vi "pointer.permute.advanced copy.vi"(8 "error in (no error)":errorcluster, 11 "TestCase in":refnum<class "TestCase.Pointer.lvclass">) -> (0 "error out":errorcluster, 2 "pass?":bool, 3 "TestCase out":refnum<class "TestCase.Pointer.lvclass">)   [LabVIEW 2016, in "TestCase.Pointer.lvclass"]
uses:
  TestCase.Pointer.lvclass
  TestCase.Pointer.lvclass/TestCase.Pointer.ctl
  Source/Classes/Pointer/Memory.Pointer.Write.0D.DBL.vi
  Source/Classes/Pointer/Memory.Pointer.Read.0D.U8.vi
  Source/Classes/Pointer/Memory.Pointer.Read.0D.U16.vi
  Source/Classes/Pointer/Memory.Pointer.Read.0D.U32.vi
  Source/Classes/Pointer/Memory.Pointer.Read.0D.U64.vi
  Source/Classes/Pointer/Memory.Pointer.lvclass
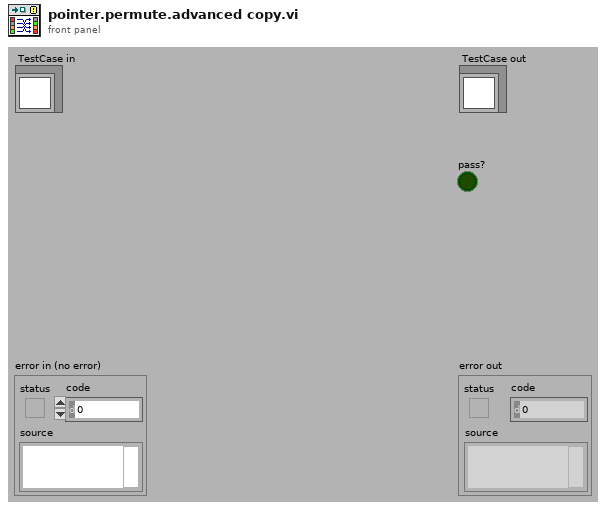
[diagram p1: front panel]
types:
  T1 = enum16{"big-endian, network order", "native, host order", "little-endian"}
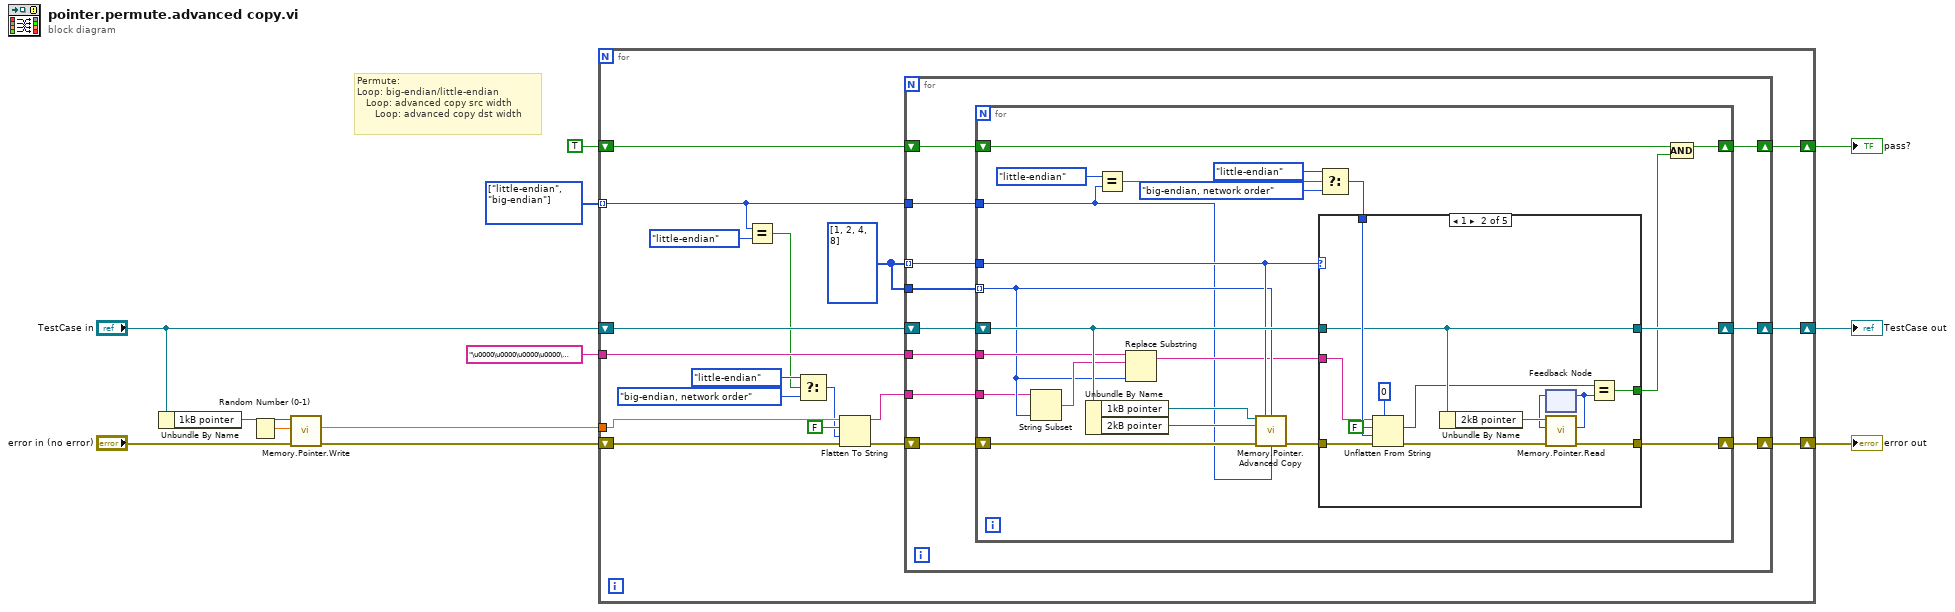
[diagram p0: block diagram]
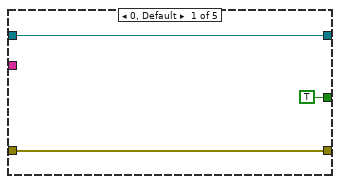
[diagram p2: hidden frame]
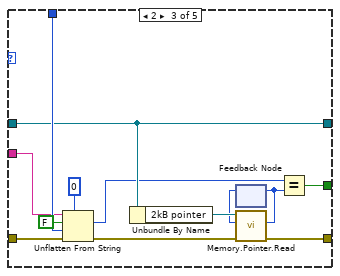
[diagram p3: hidden frame]
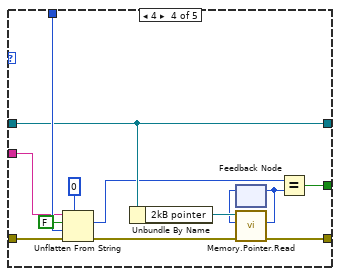
[diagram p4: hidden frame]
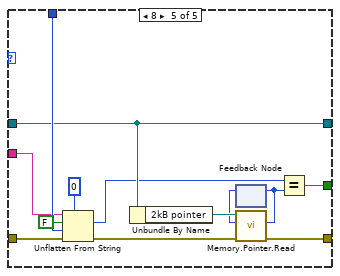
[diagram p5: hidden frame]
diagram:
  w10 = enum16{"big-endian", "little-endian"}[] [enum."little-endian", enum."big-endian"] items=["big-endian", "little-endian"] ("byte order (big-endian)")
  # "Permute:\nLoop: big-endian/little-endian\n   Loop: advanced copy src width\n      Loop: advanced copy dst width"
  n1 = Unbundle By Name("TestCase in") -> ("1kB pointer"=w9:refnum<class "Memory.Pointer.lvclass">)
  n2 = Random Number (0-1)() -> (number: 0 to 1=w8:dbl)
  n3 = call-poly "Memory.Pointer.Write.vi"("error in (no error)"="error in (no error)", "value"=w8, "Pointer in"=w9) -> ("error out"=w1:errorcluster, "value"=w2:dbl)  [unwired: 5 in, 2 out]
  n4 = for {
    shift-right: [w29] -> w12
    shift-left: w1 -> [w22]
    shift-right: [w28] -> w11
    shift-left: "TestCase in" -> [w30]
    tunnel: w10 -> [w13] mode=indexing
    shift-right: [w25] -> w4
    shift-left: TRUE -> [w26]
    tunnel: "\u0000\u0000\u0000\u0000\u0000\u0000\u0000\u0000" -> [w24]
    tunnel: w2 -> [w19]
    w27 = u64[] [1, 2, 4, 8] ("dst width")
    n5 = Equal?(x=w13, y=enum16{"big-endian", "little-endian"}."little-endian" ("byte order (big-endian)")) -> (x = y?=w15:bool)
    n6 = Select(t=T1."little-endian" ("byte order (0:big-endian, network order)"), s=w15, f=T1."big-endian, network order" ("byte order (0:big-endian, network order)")) -> (s? t:f=w16:T1)
    n7 = Flatten To String(anything=w19, prepend array or string size? (T)=FALSE, byte order (0:big-endian, network order)=w16, error in (no error)=w22) -> (data string=w20:string, error out=w21:errorcluster)  [unwired: 1 out]
    n8 = for {
      shift-right: [w38] -> w28
      shift-left: w30 -> [w40]
      shift-right: [w39] -> w29
      shift-left: w21 -> [w41]
      tunnel: w27 -> [w37] mode=indexing
      tunnel: w27 -> [w36]
      tunnel: w13 -> [w35]
      tunnel: w20 -> [w34]
      shift-right: [w32] -> w25
      shift-left: w26 -> [w33]
      tunnel: w24 -> [w31]
      n9 = for {
        shift-right: [w58] -> w38
        shift-left: w40 -> [w59]
        shift-right: [w57] -> w39
        shift-left: w41 -> [w51]
        tunnel: w37 -> [w47]
        tunnel: w36 -> [w46] mode=indexing
        tunnel: w35 -> [w42]
        tunnel: w34 -> [w45]
        shift-right: [w54] -> w32
        shift-left: w33 -> [w56]
        tunnel: w31 -> [w49]
        n10 = String Subset(string=w45, length (rest)=w46) -> (substring=w48:string)  [unwired: 1 in]
        n11 = Unbundle By Name(w59) -> ("1kB pointer"=w53:refnum<class "Memory.Pointer.lvclass">, "2kB pointer"=w52:refnum<class "Memory.Pointer.lvclass">)
        n12 = Equal?(x=enum16{"big-endian", "little-endian"}."little-endian" ("byte order (big-endian)"), y=w42) -> (x = y?=w63:bool)
        n13 = Replace Substring(2:w46, 4:w48, 5:w49) -> (1:w44:string)  [unwired: 1 in, 1 out]
        n14 = call "Memory.Pointer.Advanced Copy.vi"("src Pointer in"=w53, "dst width"=w47, "src width"=w46, "dst Pointer in"=w52, "error in (no error)"=w51, "dst byte order (little-endian)"=w42) -> ("error out"=w60:errorcluster)  [unwired: 7 in, 2 out]
        n15 = Select(t=T1."little-endian" ("byte order (0:big-endian, network order)"), s=w63, f=T1."big-endian, network order" ("byte order (0:big-endian, network order)")) -> (s? t:f=w43:T1)
        n16 = case shown="1" w47 {
          tunnel: w60 -> [w65 w79 w92 w105 w118]
          tunnel: w43 -> [_ w78 w91 w104 w117]
          tunnel: w59 -> [w66 w68 w89 w102 w115]
          tunnel: [w66 w68 w89 w102 w115] -> w58
          tunnel: [w65 w74 w86 w98 w111] -> w57
          tunnel: [TRUE w73 w85 w97 w110] -> w55
          tunnel: w44 -> [_ w71 w83 w95 w108]
          frame 0, Default {
          }
          frame 1 {
            n17 = Unflatten From String(type=u8 0, binary string=w71, data includes array or string size? (T)=FALSE, byte order (0:big-endian, network order)=w78, error in (no error)=w79) -> (value=w67:u8, error out=w75:errorcluster)  [unwired: 1 out]
            n18 = Unbundle By Name(w68) -> ("2kB pointer"=w76:refnum<class "Memory.Pointer.lvclass">)
            n19 = feedback #1() -> (w69:u8)  [unwired: 1 in]
            n20 = call-poly "Memory.Pointer.Read.vi"("error in (no error)"=w75, "value in"=w69, "Pointer in"=w76) -> ("error out"=w74:errorcluster, "value out"=w70:u8)  [unwired: 5 in, 2 out]
            n21 = feedback-in #1(w70) -> ()
            n22 = Equal?(x=w67, y=w70) -> (x = y?=w73:bool)
          }
          frame 2 {
            n23 = Unflatten From String(type=u16 0, binary string=w83, data includes array or string size? (T)=FALSE, byte order (0:big-endian, network order)=w91, error in (no error)=w92) -> (value=w82:u16, error out=w87:errorcluster)  [unwired: 1 out]
            n24 = Unbundle By Name(w89) -> ("2kB pointer"=w88:refnum<class "Memory.Pointer.lvclass">)
            n25 = feedback #2() -> (w80:u16)  [unwired: 1 in]
            n26 = call-poly "Memory.Pointer.Read.vi"("error in (no error)"=w87, "value in"=w80, "Pointer in"=w88) -> ("error out"=w86:errorcluster, "value out"=w81:u16)  [unwired: 5 in, 2 out]
            n27 = feedback-in #2(w81) -> ()
            n28 = Equal?(x=w82, y=w81) -> (x = y?=w85:bool)
          }
          frame 4 {
            n29 = Unflatten From String(type=u32 0, binary string=w95, data includes array or string size? (T)=FALSE, byte order (0:big-endian, network order)=w104, error in (no error)=w105) -> (value=w99:u32, error out=w100:errorcluster)  [unwired: 1 out]
            n30 = Unbundle By Name(w102) -> ("2kB pointer"=w101:refnum<class "Memory.Pointer.lvclass">)
            n31 = feedback #3() -> (w93:u32)  [unwired: 1 in]
            n32 = call-poly "Memory.Pointer.Read.vi"("error in (no error)"=w100, "value in"=w93, "Pointer in"=w101) -> ("error out"=w98:errorcluster, "value out"=w94:u32)  [unwired: 5 in, 2 out]
            n33 = feedback-in #3(w94) -> ()
            n34 = Equal?(x=w99, y=w94) -> (x = y?=w97:bool)
          }
          frame 8 {
            n35 = Unflatten From String(type=u64 0, binary string=w108, data includes array or string size? (T)=FALSE, byte order (0:big-endian, network order)=w117, error in (no error)=w118) -> (value=w112:u64, error out=w113:errorcluster)  [unwired: 1 out]
            n36 = Unbundle By Name(w115) -> ("2kB pointer"=w114:refnum<class "Memory.Pointer.lvclass">)
            n37 = feedback #4() -> (w106:u64)  [unwired: 1 in]
            n38 = call-poly "Memory.Pointer.Read.vi"("error in (no error)"=w113, "value in"=w106, "Pointer in"=w114) -> ("error out"=w111:errorcluster, "value out"=w107:u64)  [unwired: 5 in, 2 out]
            n39 = feedback-in #4(w107) -> ()
            n40 = Equal?(x=w112, y=w107) -> (x = y?=w110:bool)
          }
        }
        n41 = Compound Arithmetic op=AND(w56, w55) -> (w54:bool)
      }
    }
  }
  "error out" <- w12
  "TestCase out" <- w11
  "pass?" <- w4
